vi "write galvo tasks.vi"(8 "error in (no error)":errorcluster, 11 "Waveform in":refnum<class "Waveform.lvclass">) -> (0 "error out":errorcluster, 3 "Waveform out":refnum<class "Waveform.lvclass">)   [LabVIEW 2012, in "Waveform.lvclass"]
uses:
  Waveform.lvclass
  Waveform.lvclass/Waveform.ctl
  <vilib>/DAQmx/write.llb/DAQmx Write (Analog 1D Wfm NChan NSamp).vi
  <vilib>/DAQmx/miscellaneous.llb/DAQmx Fill In Error Info.vi
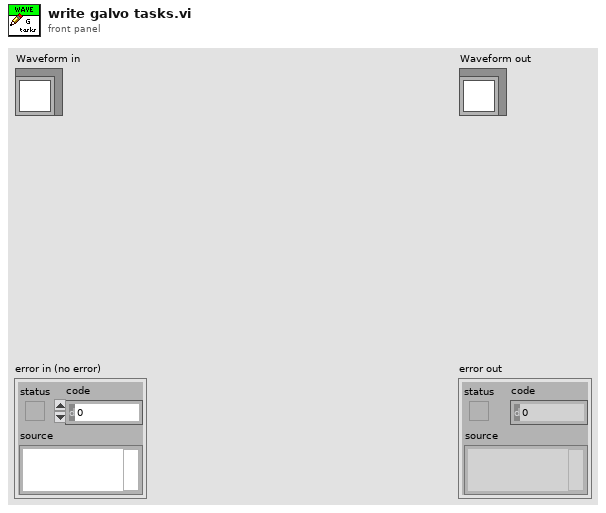
[diagram p1: front panel]
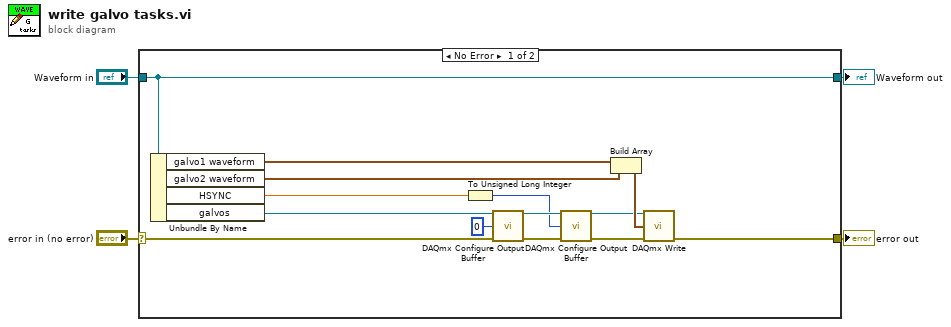
[diagram p0: block diagram]
diagram:
  n1 = case shown="No Error" "error in (no error)" {
    selector: "error in (no error)" -> [w6 w20]
    tunnel: [w15 w20] -> w3
    tunnel: [w18 w19] -> w1
    tunnel: "Waveform in" -> [w18 w19]
    frame No Error {
      n2 = Unbundle By Name(w18) -> ("galvo1 waveform"=w9:waveform(dbl), "galvo2 waveform"=w17:waveform(dbl), "HSYNC"=w11:dbl, "galvos"=w5:refnum<k21>)
      n3 = To Unsigned Long Integer(number=w11) -> (unsigned 32bit integer=w7:u32)
      n4 = call <vilib>:"DAQmx Configure Output Buffer.vi"("task/channels in"=w5, "buffer size (in samples per channel)"=u32 0, "error in"=w6) -> ("task out"=w8:refnum<k21>, "error out"=w13:errorcluster)  [unwired: 11 in]
      n5 = call <vilib>:"DAQmx Configure Output Buffer.vi"("task/channels in"=w8, "buffer size (in samples per channel)"=w7, "error in"=w13) -> ("task out"=w10:refnum<k21>, "error out"=w12:errorcluster)  [unwired: 11 in]
      n6 = Build Array(w9, w17) -> (w16:waveform(dbl)[])
      n7 = call-poly <vilib>:"DAQmx Write.vi"("task/channels in"=w10, "data"=w16, "error in"=w12) -> ("error out"=w15:errorcluster)  [unwired: 10 in, 2 out]
    }
    frame Error {
    }
  }
  "error out" <- w3
  "Waveform out" <- w1
